vi "Simulator.vi"() -> ()   [LabVIEW 2017]
uses:
  <vilib>/DAQmx/read.llb/DAQmx Read (Digital 1D Bool NChan 1Samp 1Line).vi
  <vilib>/DAQmx/write.llb/DAQmx Write (Analog 1D DBL NChan 1Samp).vi
  <vilib>/DAQmx/create/channels.llb/DAQmx Create Channel (AO-Voltage-Basic).vi
  <vilib>/DAQmx/miscellaneous.llb/DAQmx Fill In Error Info.vi
  <vilib>/DAQmx/create/channels.llb/DAQmx Create Channel (DI-Digital Input).vi
  Global_simulator.vi
  <vilib>/Utility/file.llb/Write Delimited Spreadsheet (DBL).vi
  <vilib>/Utility/file.llb/Write Delimited Spreadsheet (string).vi
panel:
  out "Y 2":dbl[](array[numeric])
  out "Y":dbl[](array[numeric])
  out "Waveform Chart 2":waveform(dbl)(graph)
  out "Waveform Chart":waveform(dbl)(graph)
  in  "stop":bool
  out "data 3":bool[](array[boolean])
  out "x+y":i16
  out "element":bool
  out "element 2":bool
  out "x+y 2":i16
  in  "File Path Control":path
  in  "delta(ms)":i32
  in  "Off Time(ms)":i32
  in  "No of Rotation":i32
  in  "Dwell Time(ms)":i32
  out "Square":waveform(dbl)[](graph)
  in  "Frequency(Hz)":dbl=20.0 caption="Frequency"
  in  "Duty Cycle (%)":dbl=50.0
  # "Signal Generator"
  # "Test Properties"
  # "Signal Properties"
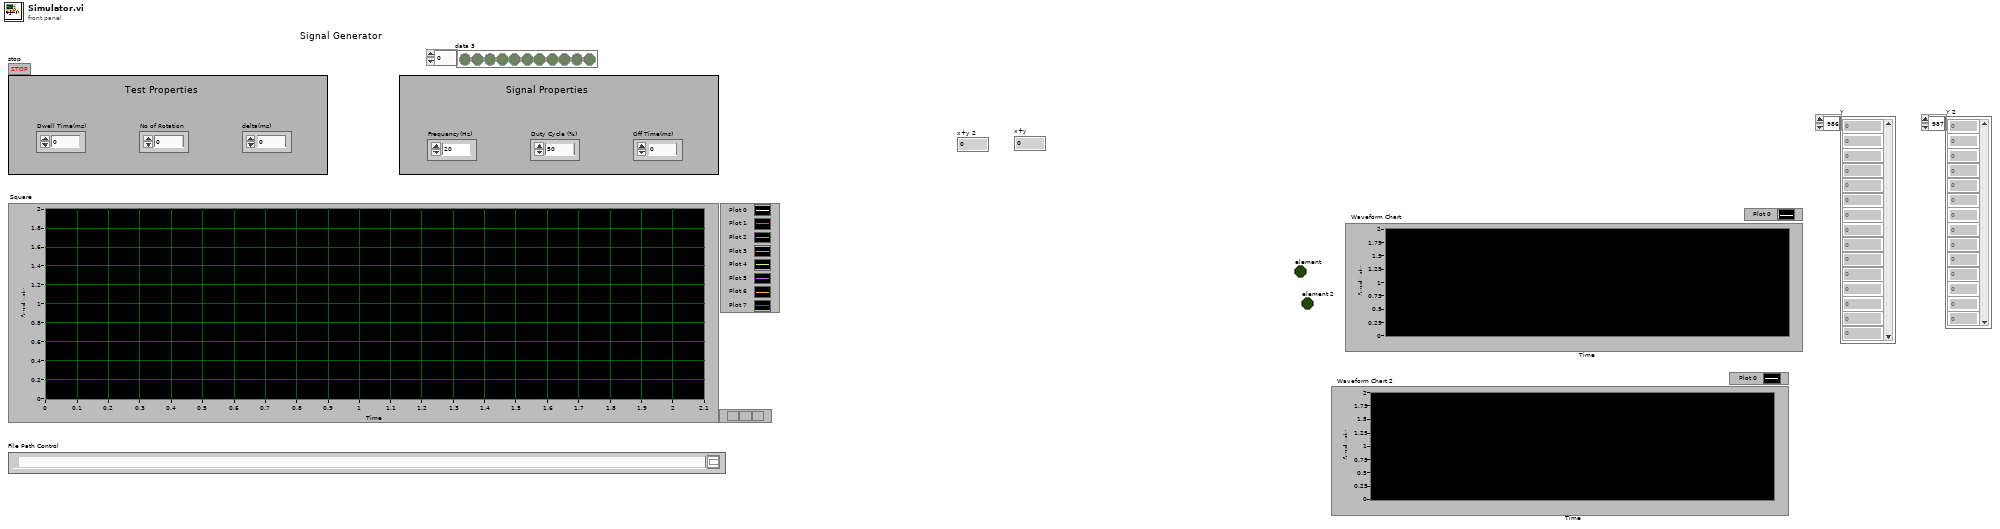
[diagram p1: front panel]
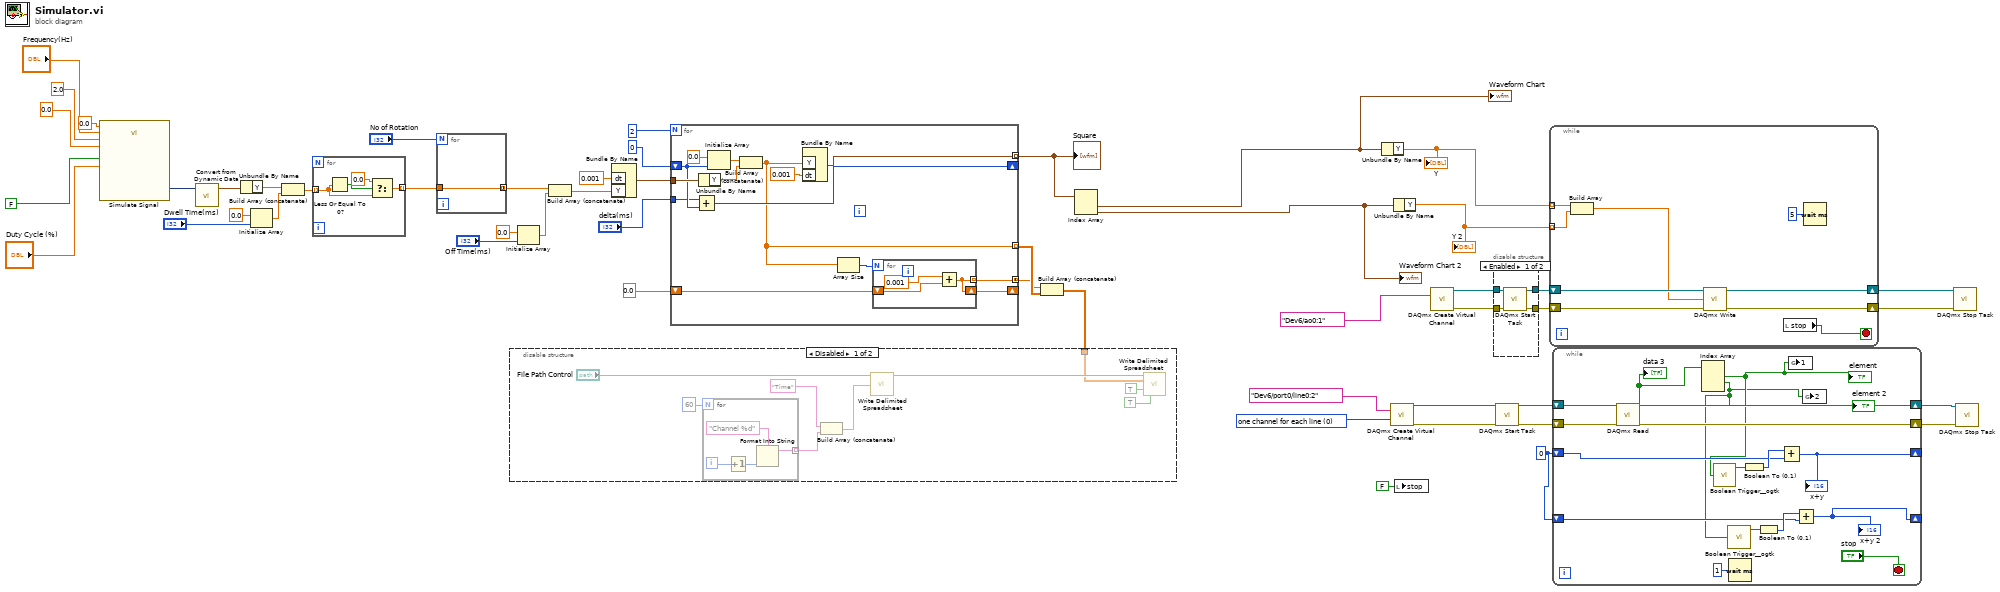
[diagram p0: block diagram]
diagram:
  w6 = 0 items=["one channel for each line", "one channel for all lines"] ("line grouping")
  w5 = i16 0
  n1 = call "Simulate Signal"("Offset"=0.0, "Duty Cycle (%)"="Duty Cycle (%)", "Reset Signal"=FALSE, "Frequency"="Frequency(Hz)", "Amplitude"=2.0, "Phase"=0.0) -> ("Square"=w45:dynamicdata)  [unwired: 8 in, 1 out]
  n2 = call "Convert from Dynamic Data"("Dynamic Data Type"=w45) -> ("Waveform"=w41:waveform(dbl))  [unwired: 3 in]
  n3 = Unbundle By Name(w41) -> ("Y"=w40:dbl[])
  n4 = Initialize Array(0.0 ("element"), "Dwell Time(ms)") -> (w39:dbl[])
  n5 = Build Array (concatenate)(w40, w39) -> (w37:dbl[])
  n6 = for {
    tunnel: w37 -> [w53] mode=indexing
    tunnel: [w52] -> w36 mode=indexing
    n7 = Less Or Equal To 0?(x=w53) -> (x <= 0?=w55:bool)
    n8 = Select(t=0.0, s=w55, f=w53) -> (s? t:f=w52:dbl)
  }
  n9 = for {
    N: "No of Rotation" -> [_]
    tunnel: w36 -> [w56]
    tunnel: [w56] -> w33 mode=concatenating
  }
  n10 = Initialize Array(0.0 ("element"), "Off Time(ms)") -> (w32:dbl[])
  n11 = Build Array (concatenate)(w33, w32) -> (w31:dbl[])
  n12 = Bundle By Name("dt"=0.001, "Y"=w31) -> (w29:waveform(dbl))  [unwired: 1 in]
  n13 = for {
    N: 2 -> [_]
    tunnel: w29 -> [w70]
    shift-right: [w66] -> _
    shift-left: 0 -> [w68]
    tunnel: "delta(ms)" -> [w67]
    tunnel: [w63] -> w3 mode=indexing
    tunnel: [w60] -> w26 mode=indexing
    tunnel: [w59] -> w25 mode=concatenating
    shift-right: [w57] -> _
    shift-left: 0.0 ("dt") -> [w58]
    n14 = Add(x=w67, y=w68) -> (x+y=w66:i32)
    n15 = Unbundle By Name(w70) -> ("Y"=w65:dbl[])
    n16 = Initialize Array(0.0 ("element"), w68) -> (w64:dbl[])
    n17 = Build Array (concatenate)(w64, w65) -> (w60:dbl[])
    n18 = Bundle By Name("Y"=w60, "dt"=0.001) -> (w63:waveform(dbl))  [unwired: 1 in]
    n19 = Array Size(array=w60) -> (size(s)=w61:i32)
    n20 = for {
      N: w61 -> [_]
      tunnel: [w72] -> w59 mode=indexing
      shift-right: [w72] -> w57
      shift-left: w58 -> [w73]
      n21 = Add(x=0.001 ("dt"), y=w73) -> (x+y=w72:dbl)
    }
  }
  "Square" <- w3
  n22 = Build Array (concatenate)(w25, w26) -> (w24:dbl[][])
  n23 = disable-structure shown="Disabled" {
    disable-tunnel: w24 -> [w77 _]
    frame Disabled {
      n24 = for {
        N: 60 -> [_]
        tunnel: [w83] -> w75 mode=indexing
        i -> [w84]
        n25 = Increment(x=w84) -> (x+1=w85:i32)
        n26 = Format Into String(format string="Channel %d", w85) -> (resulting string=w83:string)  [unwired: 2 in, 1 out]
      }
      n27 = Build Array (concatenate)("Time", w75) -> (w74:string[])
      n28 = call-poly <vilib>:"Write Delimited Spreadsheet.vi"("file path (dialog if empty)"="File Path Control", "1D data"=w74) -> ("new file path (Not A Path if cancelled)"=w81:path)  [unwired: 12 in, 1 out]
      n29 = call-poly <vilib>:"Write Delimited Spreadsheet.vi"("file path (dialog if empty)"=w81, "2D data"=w77, "append to file? (new file:F)"=TRUE, "transpose? (no:F)"=TRUE) -> ()  [unwired: 10 in, 2 out]
    }
    frame Enabled {
    }
  }
  n30 = Index Array(array=w3) -> (element #1=w2:waveform(dbl), element #2=w1:waveform(dbl))  [unwired: 2 in]
  "Waveform Chart" <- w2
  "Waveform Chart 2" <- w1
  n31 = Unbundle By Name(w2) -> ("Y"=w8:dbl[])
  "Y" <- w8
  n32 = call-poly <vilib>:"DAQmx Create Virtual Channel.vi"("lines"=tag "Dev6/port0/line0:2", "line grouping"=w6) -> ("task out"=w13:refnum<k21>, "error out"=w11:errorcluster)  [unwired: 12 in]
  n33 = Unbundle By Name(w1) -> ("Y"=w7:dbl[])
  "Y 2" <- w7
  n34 = local write "stop"(FALSE ("stop")) -> ()
  n35 = call-poly <vilib>:"DAQmx Create Virtual Channel.vi"("physical channels"=tag "Dev6/ao0:1") -> ("task out"=w18:refnum<k21>, "error out"=w17:errorcluster)  [unwired: 13 in]
  n36 = disable-structure shown="Enabled" {
    disable-tunnel: [w90 w91] -> w20
    disable-tunnel: [w89 _] -> w19
    disable-tunnel: w18 -> [w88 w91]
    disable-tunnel: w17 -> [w87 _]
    frame Enabled {
      n37 = call <vilib>:"DAQmx Start Task.vi"("task/channels in"=w88, "error in"=w87) -> ("task out"=w90:refnum<k21>, "error out"=w89:errorcluster)  [unwired: 12 in]
    }
    frame Disabled {
    }
  }
  n38 = call <vilib>:"DAQmx Start Task.vi"("task/channels in"=w13, "error in"=w11) -> ("task out"=w12:refnum<k21>, "error out"=w10:errorcluster)  [unwired: 12 in]
  n39 = while {
    shift-right: [w100] -> w22
    shift-left: w20 -> [w98]
    shift-right: [w99] -> w21
    shift-left: w19 -> [w97]
    tunnel: w8 -> [w95] mode=indexing
    tunnel: w7 -> [w93] mode=indexing
    stop <- w92 stop-if-true
    n40 = Build Array(w95, w93) -> (w94:dbl[])
    n41 = call-poly <vilib>:"DAQmx Write.vi"("task/channels in"=w98, "data"=w94, "error in"=w97) -> ("task out"=w100:refnum<k21>, "error out"=w99:errorcluster)  [unwired: 10 in, 1 out]
    n42 = local read "stop"() -> (w92:bool)
    n43 = Wait (ms)(milliseconds to wait=u32 5) -> ()  [unwired: 1 out]
  }
  n44 = while {
    shift-right: [w117] -> w16
    shift-left: w12 -> [w115]
    shift-right: [w116] -> w15
    shift-left: w10 -> [w114]
    shift-right: [w110] -> _
    shift-left: w5 -> [w109]
    shift-right: [w103] -> _
    shift-left: w5 -> [w104]
    stop <- "stop" stop-if-true
    n45 = call-poly <vilib>:"DAQmx Read.vi"("task/channels in"=w115, "error in"=w114) -> ("task out"=w117:refnum<k21>, "data"=w107:bool[], "error out"=w116:errorcluster)  [unwired: 11 in]
    "data 3" <- w107
    n46 = Index Array(array=w107) -> (element #1=w102:bool, element #2=w101:bool)  [unwired: 3 in, 1 out]
    "element" <- w102
    "element 2" <- w101
    n47 = call <userlib>:"Boolean Trigger__ogtk.vi"("Boolean Input"=w102) -> ("Rising Edge"=w108:bool)  [unwired: 1 in, 1 out]
    n48 = call <userlib>:"Boolean Trigger__ogtk.vi"("Boolean Input"=w101) -> ("Rising Edge"=w106:bool)  [unwired: 1 in, 1 out]
    n49 = Wait (ms)(milliseconds to wait=u32 1) -> ()  [unwired: 1 out]
    n50 = Boolean To (0,1)(Boolean=w108) -> (0, 1=w111:i16)
    n51 = Boolean To (0,1)(Boolean=w106) -> (0, 1=w105:i16)
    n52 = Add(x=w111, y=w109) -> (x+y=w110:i16)
    "x+y" <- w110
    n53 = global write "Global_simulator.vi" "1"(w102) -> ()
    n54 = Add(x=w105, y=w104) -> (x+y=w103:i16)
    "x+y 2" <- w103
    n55 = global write "Global_simulator.vi" "2"(w101) -> ()
  }
  n56 = call <vilib>:"DAQmx Stop Task.vi"("task/channels in"=w22, "error in"=w21) -> ()  [unwired: 12 in, 2 out]
  n57 = call <vilib>:"DAQmx Stop Task.vi"("task/channels in"=w16, "error in"=w15) -> ()  [unwired: 12 in, 2 out]
